vi "Read Enable.vi"(11 "Effect Interface in":refnum<class "Effect Interface.lvclass">) -> (2 "Enable":bool, 3 "Effect Interface out":refnum<class "Effect Interface.lvclass">)   [LabVIEW 2019, in "Effect Interface.lvlib" / "Effect Interface.lvclass"]
uses:
  Effect Interface.lvclass
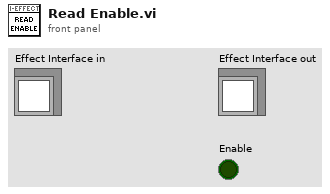
[diagram p1: front panel]
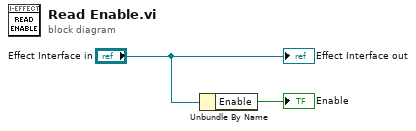
[diagram p0: block diagram]
diagram:
  n1 = Unbundle By Name("Effect Interface in") -> ("Enable"=→"Enable":bool)
  "Effect Interface out" <- "Effect Interface in"
